vi "loadSummaryReport.vi"(10 "path":path=path "C:/temp/summary") -> (0 "error out":errorcluster, 2 "Files":string)   [LabVIEW 2012]
uses:
  <vilib>/addons/database/Connection.llb/DB Tools Open Connec (Path).vi
  <vilib>/addons/database/NI_Database_API.lvlib
panel:
  in  "input cluster 2":T1
  out "concatenated string":string
  out "concatenated string 2":string
  out "trimmed string":string
  out "filenames":string[](array[string])
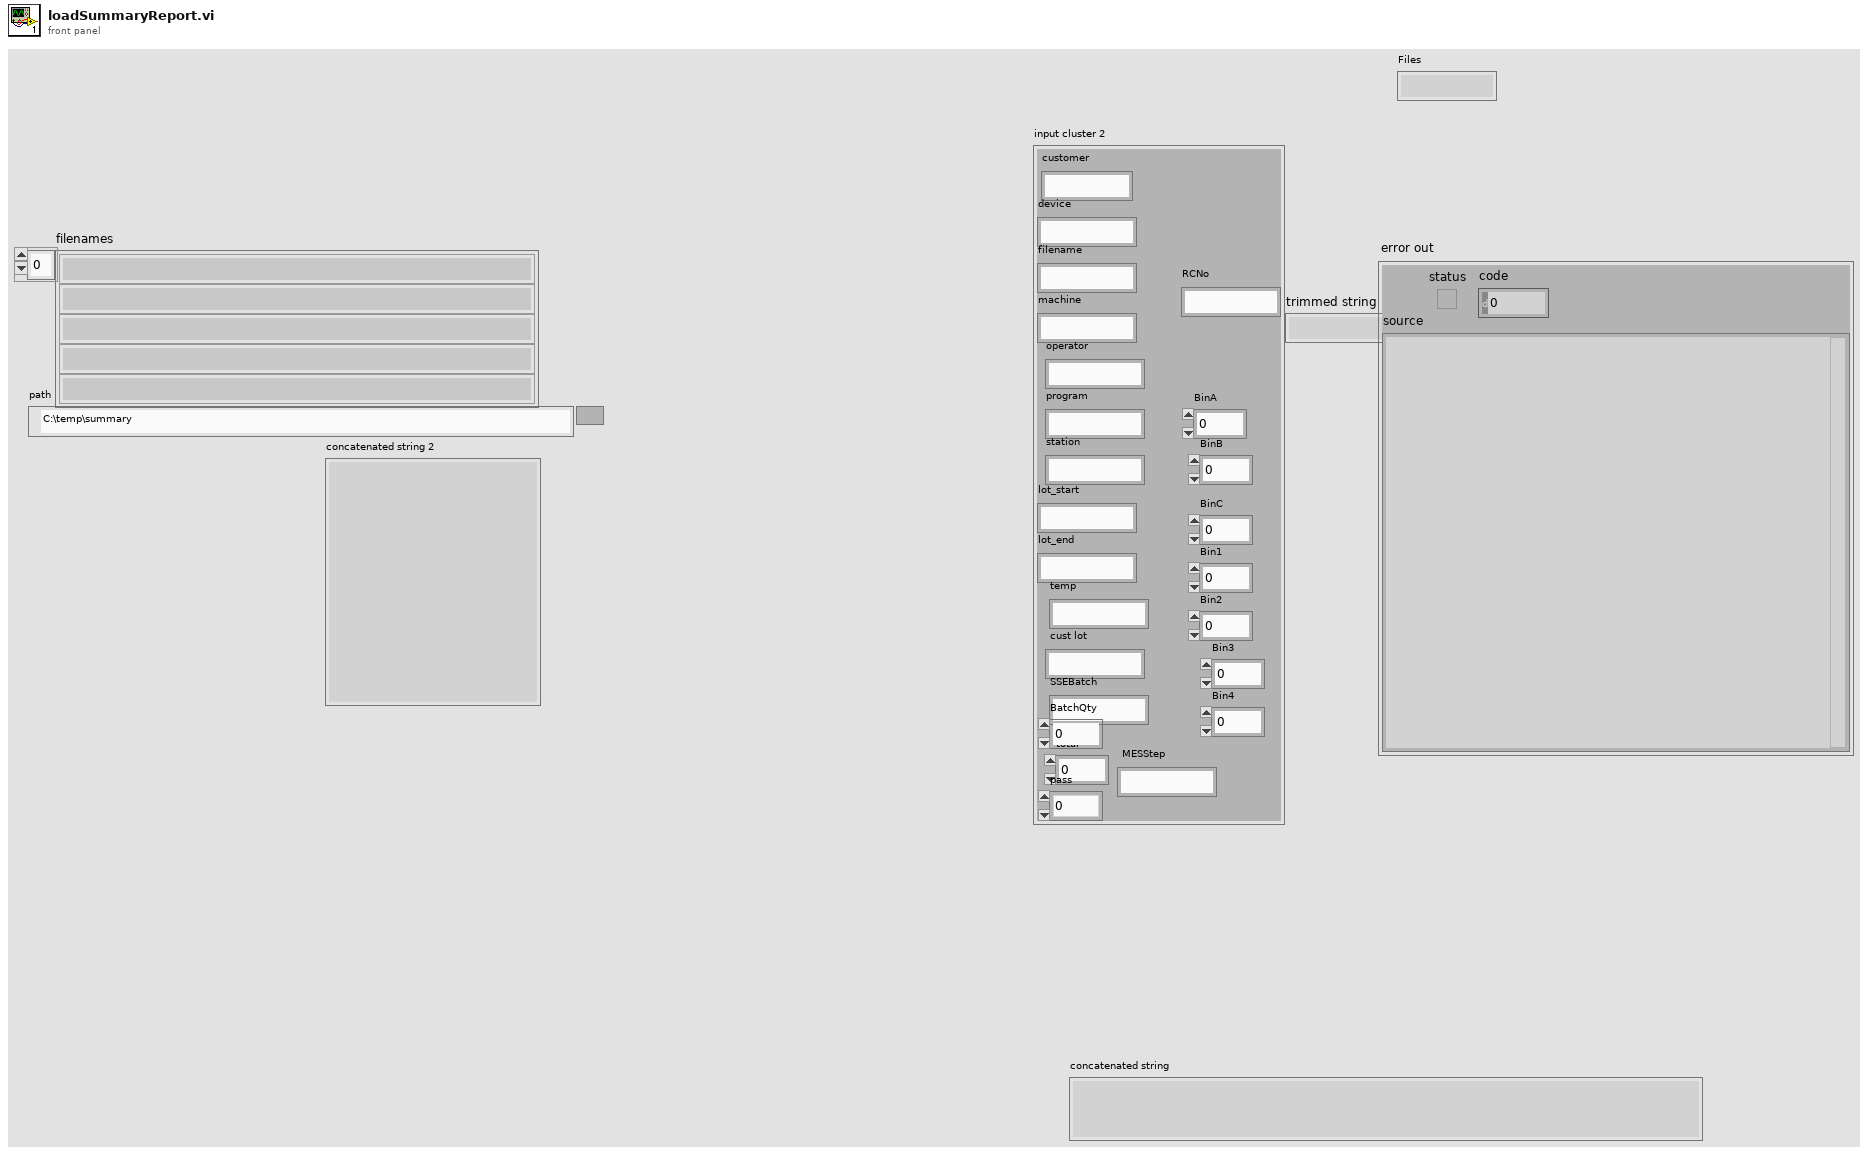
[diagram p1: front panel]
types:
  T1 = cluster{"customer":string, "device":string, "filename":string, "RCNo":string, "machine":string, "operator":string, "program":string, "station":string, "lot_start":string, "lot_end":string, "temp":string, "cust lot":string, "SSEBatch":string, "BatchQty":dbl, "total":dbl, "pass":dbl, "BinA":dbl, "BinB":dbl, "BinC":dbl, "Bin1":dbl, "Bin2":dbl, "Bin3":dbl, "Bin4":dbl, "MESStep":string}
  T2 = typedef "NI_Database_API.lvlib/Conn ObjectReference.ctl" = refnum<k1>
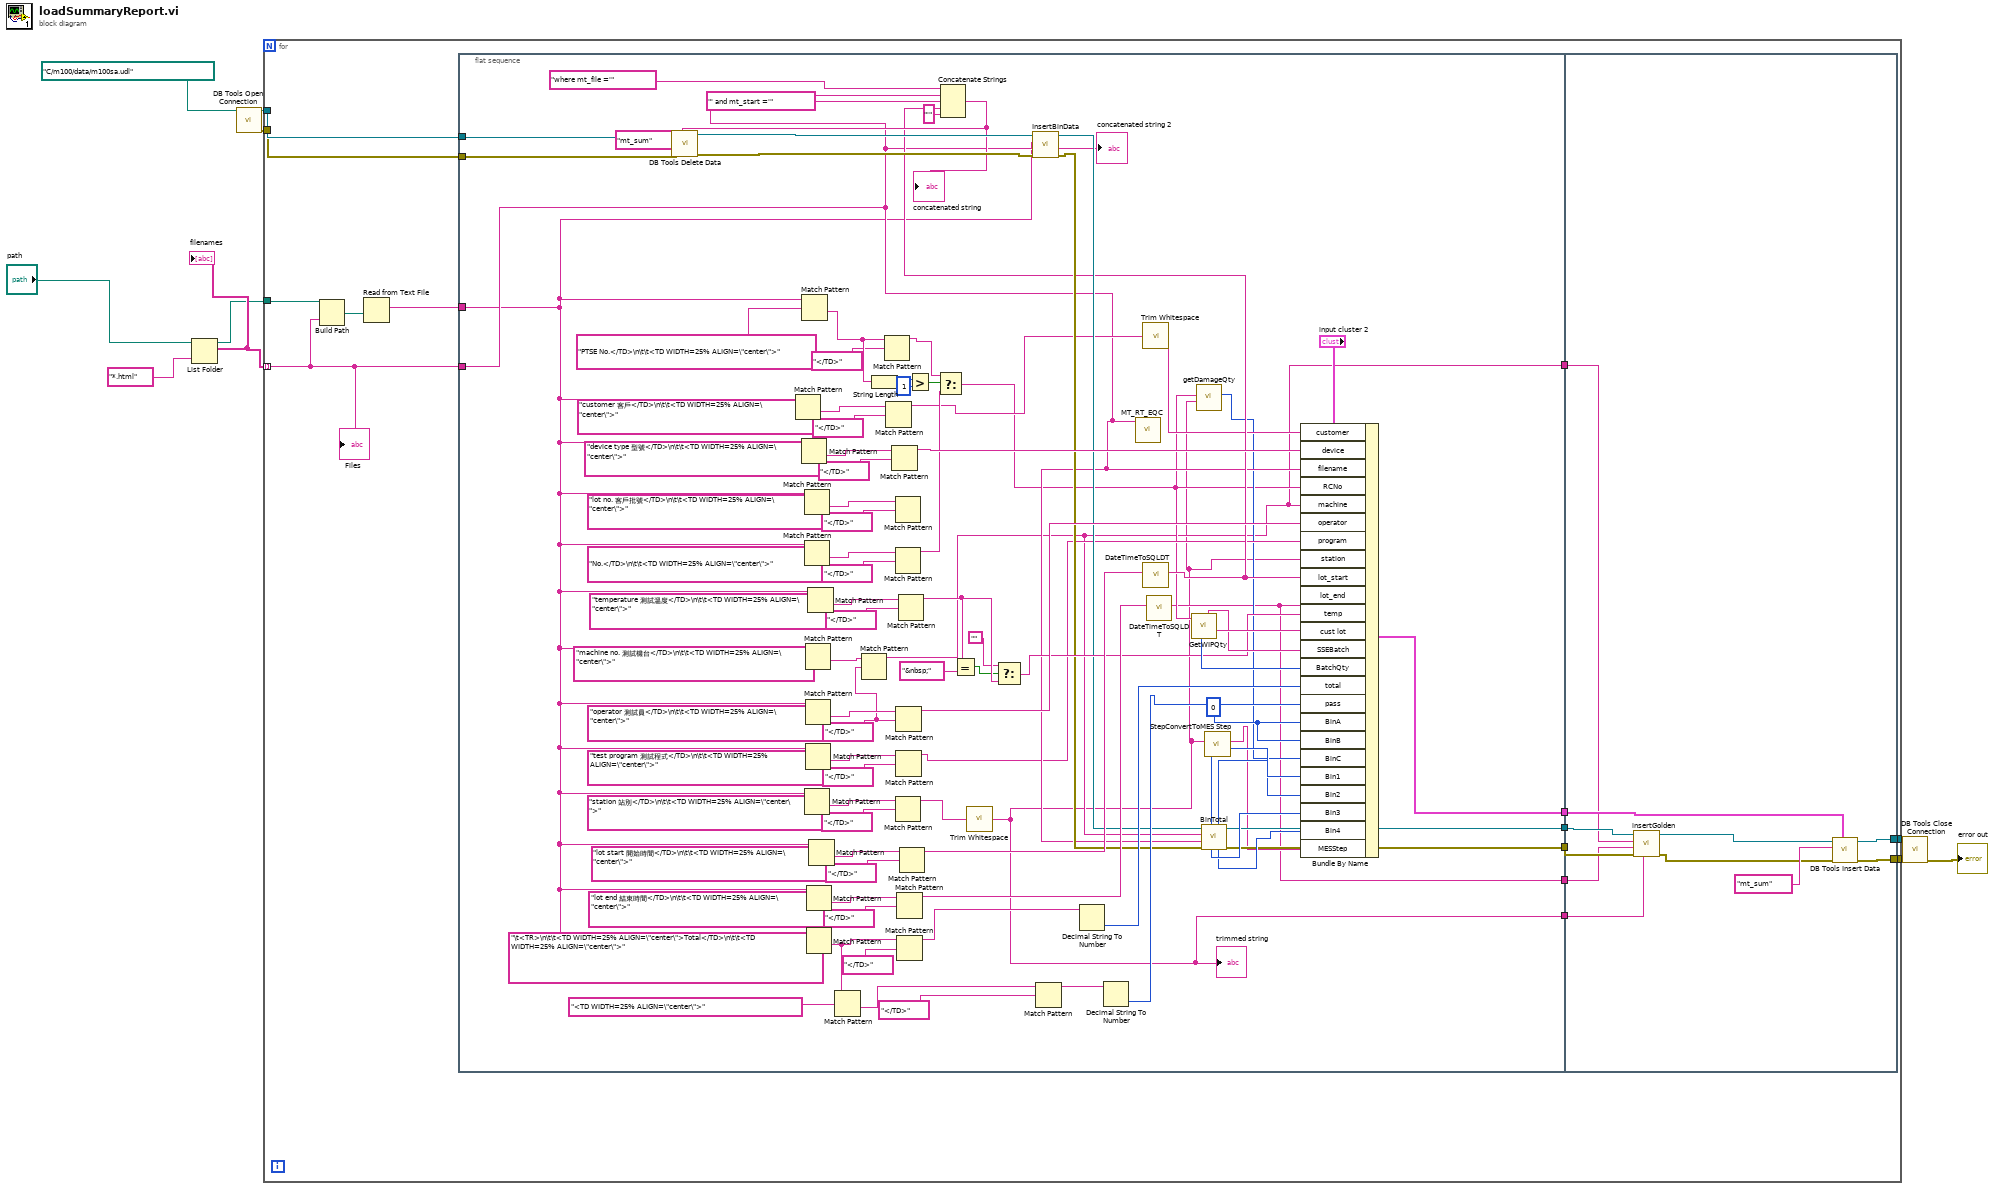
[diagram p0: block diagram]
diagram:
  n1 = List Folder(path="path", pattern="*.html") -> (path out=w8:path, filenames=w9:string[])  [unwired: 2 in, 2 out]
  "filenames" <- w9
  n2 = call-poly <vilib>:"DB Tools Open Connection.vi"("connection information"=path "C:/m100/data/m100sa.udl") -> ("error out"=w4:errorcluster, "connection reference"=w5:T2)  [unwired: 7 in]
  n3 = for {
    tunnel: w9 -> [w14] mode=indexing
    tunnel: w8 -> [w23]
    tunnel: w5 -> [w22]
    tunnel: w4 -> [w21]
    tunnel: [w17] -> w3
    tunnel: [w16] -> w2
    n4 = Build Path(base path=w23, name or relative path=w14) -> (appended path=w24:path)
    n5 = Read from Text File(file (use dialog)=w24) -> (text=w20:string)  [unwired: 3 in, 3 out]
    n6 = flat-sequence {
      tunnel: w22 -> [w43]
      tunnel: w21 -> [w42]
      tunnel: w20 -> [w30]
      tunnel: [w50] -> w19
      tunnel: [w49] -> w18
      tunnel: [w37] -> w15
      tunnel: w14 -> [w33]
      tunnel: [w27] -> w13
      tunnel: [w26] -> w12
      tunnel: [w25] -> w11
      tunnel: w19 -> [w126]
      tunnel: w18 -> [w127]
      tunnel: [w130] -> w17
      tunnel: [w129] -> w16
      tunnel: w15 -> [w131]
      tunnel: w13 -> [w123]
      tunnel: w12 -> [w122]
      tunnel: w11 -> [w121]
      frame #0 {
        w48 = 0
        w57 = "</TD>" ("regular expression")
        n7 = Match Pattern(string=w30, regular expression="customer 客戶</TD>\n\t\t<TD WIDTH=25% ALIGN=\"center\">") -> (after substring=w119:string)  [unwired: 1 in, 3 out]
        n8 = Match Pattern(string=w30, regular expression="device type 型號</TD>\n\t\t<TD WIDTH=25% ALIGN=\"center\">") -> (after substring=w116:string)  [unwired: 1 in, 3 out]
        n9 = Match Pattern(string=w30, regular expression="PTSE No.</TD>\n\t\t<TD WIDTH=25% ALIGN=\"center\">") -> (after substring=w79:string)  [unwired: 1 in, 3 out]
        n10 = Match Pattern(string=w30, regular expression="lot no. 客戶批號</TD>\n\t\t<TD WIDTH=25% ALIGN=\"center\">") -> (after substring=w113:string)  [unwired: 1 in, 3 out]
        n11 = Match Pattern(string=w30, regular expression="No.</TD>\n\t\t<TD WIDTH=25% ALIGN=\"center\">") -> (after substring=w110:string)  [unwired: 1 in, 3 out]
        n12 = Match Pattern(string=w30, regular expression="station 站別</TD>\n\t\t<TD WIDTH=25% ALIGN=\"center\">") -> (after substring=w99:string)  [unwired: 1 in, 3 out]
        n13 = Match Pattern(string=w30, regular expression="machine no. 測試機台</TD>\n\t\t<TD WIDTH=25% ALIGN=\"center\">") -> (after substring=w58:string)  [unwired: 1 in, 3 out]
        n14 = Match Pattern(string=w30, regular expression="operator 測試員</TD>\n\t\t<TD WIDTH=25% ALIGN=\"center\">") -> (after substring=w104:string)  [unwired: 1 in, 3 out]
        n15 = Match Pattern(string=w30, regular expression="test program 測試程式</TD>\n\t\t<TD WIDTH=25% ALIGN=\"center\">") -> (after substring=w102:string)  [unwired: 1 in, 3 out]
        n16 = Match Pattern(string=w30, regular expression="lot end 結束時間</TD>\n\t\t<TD WIDTH=25% ALIGN=\"center\">") -> (after substring=w93:string)  [unwired: 1 in, 3 out]
        n17 = Match Pattern(string=w30, regular expression="\t<TR>\n\t\t<TD WIDTH=25% ALIGN=\"center\">Total</TD>\n\t\t<TD WIDTH=25% ALIGN=\"center\">") -> (after substring=w89:string)  [unwired: 1 in, 3 out]
        n18 = Match Pattern(string=w30, regular expression="temperature 測試溫度</TD>\n\t\t<TD WIDTH=25% ALIGN=\"center\">") -> (after substring=w107:string)  [unwired: 1 in, 3 out]
        n19 = Match Pattern(string=w30, regular expression="lot start 開始時間</TD>\n\t\t<TD WIDTH=25% ALIGN=\"center\">") -> (after substring=w96:string)  [unwired: 1 in, 3 out]
        n20 = Match Pattern(string=w89, regular expression="<TD WIDTH=25% ALIGN=\"center\">") -> (after substring=w86:string)  [unwired: 1 in, 3 out]
        n21 = Match Pattern(string=w58, regular expression=w57) -> (before substring=w27:string)  [unwired: 1 in, 3 out]
        n22 = String Length(string=w79) -> (length=w77:i32)
        n23 = Match Pattern(string=w79, regular expression="</TD>") -> (before substring=w75:string)  [unwired: 1 in, 3 out]
        n24 = Match Pattern(string=w119, regular expression="</TD>") -> (before substring=w36:string)  [unwired: 1 in, 3 out]
        n25 = Match Pattern(string=w116, regular expression="</TD>") -> (before substring=w83:string)  [unwired: 1 in, 3 out]
        n26 = Match Pattern(string=w113, regular expression="</TD>") -> ()  [unwired: 1 in, 4 out]
        n27 = Match Pattern(string=w110, regular expression="</TD>") -> (before substring=w74:string)  [unwired: 1 in, 3 out]
        n28 = Match Pattern(string=w99, regular expression="</TD>") -> (before substring=w34:string)  [unwired: 1 in, 3 out]
        n29 = Match Pattern(string=w104, regular expression=w57) -> (before substring=w82:string)  [unwired: 1 in, 3 out]
        n30 = Match Pattern(string=w102, regular expression="</TD>") -> (before substring=w32:string)  [unwired: 1 in, 3 out]
        n31 = Match Pattern(string=w93, regular expression="</TD>") -> (before substring=w72:string)  [unwired: 1 in, 3 out]
        n32 = Match Pattern(string=w89, regular expression="</TD>") -> (before substring=w85:string)  [unwired: 1 in, 3 out]
        n33 = Match Pattern(string=w107, regular expression="</TD>") -> (before substring=w61:string)  [unwired: 1 in, 3 out]
        n34 = Match Pattern(string=w96, regular expression="</TD>") -> (before substring=w73:string)  [unwired: 1 in, 3 out]
        n35 = Greater?(x=w77, y=1) -> (0:w78:bool)
        n36 = Select(t=w75, s=w78, f=w74) -> (s? t:f=w28:string)
        n37 = Equal?(x=w61, y="&nbsp;") -> (x = y?=w60:bool)
        n38 = call <vilib>:"Trim Whitespace.vi"("string"=w34) -> ("trimmed string"=w25:string)  [unwired: 1 in]
        "trimmed string" <- w25
        n39 = Select(t="", s=w60, f=w61) -> (s? t:f=w62:string)
        n40 = Match Pattern(string=w86, regular expression="</TD>") -> (before substring=w81:string)  [unwired: 1 in, 3 out]
        n41 = Decimal String To Number(string=w85) -> (number=w69:i32)  [unwired: 2 in, 1 out]
        n42 = Decimal String To Number(string=w81) -> (number=w70:i32)  [unwired: 2 in, 1 out]
        n43 = call "MT_RT_EQC.vi"("input string"=w33) -> ()  [unwired: 6 in, 5 out]
        n44 = call <vilib>:"Trim Whitespace.vi"("string"=w36) -> ("trimmed string"=w35:string)  [unwired: 1 in]
        n45 = call "DateTimeToSQLDT.vi"("DateTimeString"=w73) -> ("SQLDateTime"=w39:string)  [unwired: 10 in]
        n46 = Concatenate Strings("where mt_file ='" ("SQL query"), w33, "' and mt_start ='" ("string"), w39, "'" ("string")) -> (w40:string)
        "concatenated string" <- w40
        n47 = call <vilib>:"DB Tools Delete Data.vi"("condition"=w40, "error in (no error)"=w42, "table"="mt_sum", "connection reference"=w43) -> ("error out"=w44:errorcluster, "connection reference out"=w45:T2)  [unwired: 6 in]
        n48 = call "InsertBinData.vi"("error in (no error)"=w44, "FileName"=w33, "string"=w30, "connection reference"=w45) -> ("error out"=w52:errorcluster, "concatenated string"=→"concatenated string 2":string, "connection reference out"=w51:T2)  [unwired: 5 in]
        n49 = call "DateTimeToSQLDT.vi"("DateTimeString"=w72) -> ("SQLDateTime"=w26:string)  [unwired: 10 in]
        n50 = call "GetWIPQty.vi"("Lotno"=w28) -> ("lotno"=w71:string, "SSEBATCH"=w67:string, "BATCHQTY"=w68:i32)  [unwired: 2 in, 6 out]
        n51 = call "getDamageQty.vi"("Step"=w25, "RCNo"=w28) -> ("Damage"=w31:i32)  [unwired: 9 in]
        n52 = call "BinTotal.vi"("error out 2"=w52, "fileName"=w33, "machine"=w27, "connection reference"=w51) -> ("error out"=w49:errorcluster, "connection reference 2"=w50:T2, "bin4"=w53:i32, "bin2"=w55:i32, "bin3"=w54:i32, "bin1"=w56:i32)  [unwired: 2 in]
        n53 = call "StepConvertToMES Step.vi"("Step"=w25) -> ("MES Step"=w38:string)  [unwired: 10 in]
        n54 = Bundle By Name(cluster="input cluster 2", "customer"=w35, "device"=w83, "filename"=w33, "RCNo"=w28, "machine"=w27, "operator"=w82, "program"=w32, "station"=w25, "lot_start"=w39, "lot_end"=w26, "temp"=w62, "cust lot"=w71, "SSEBatch"=w67, "BatchQty"=w68, "total"=w69, "pass"=w70, "BinA"=w48, "BinB"=w48, "BinC"=w31, "Bin1"=w56, "Bin2"=w55, "Bin3"=w54, "Bin4"=w53, "MESStep"=w38) -> (w37:T1)
      }
      frame #1 {
        n55 = call "insertGolden.vi"("Station"=w121, "error in (no error)"=w127, "trans_time"=w122, "machine"=w123, "connection reference"=w126) -> ("error out"=w125:errorcluster, "connection reference 2"=w124:T2)  [unwired: 5 in]
        n56 = call <vilib>:"DB Tools Insert Data.vi"("data"=w131, "error in (no error)"=w125, "table"="mt_sum", "connection reference"=w124) -> ("error out"=w129:errorcluster, "connection reference out"=w130:T2)  [unwired: 6 in]
      }
    }
    "Files" <- w14
  }
  n57 = call <vilib>:"DB Tools Close Connection.vi"("error in (no error)"=w2, "connection reference"=w3) -> ("error out"=→"error out":errorcluster)  [unwired: 5 in]
